vi "test.vi"() -> ()   [LabVIEW 2016]
panel:
  out "decimal integer string":string
  in  "number":i32
  in  "width (-)":i16
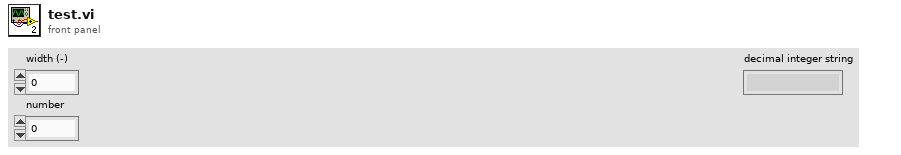
[diagram p1: front panel]
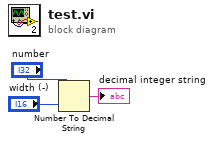
[diagram p0: block diagram]
diagram:
  n1 = Number To Decimal String(number="number", width (-)="width (-)") -> (decimal integer string=→"decimal integer string":string)
